vi "IsEmptyNextRecordListCtrl.vi"(11 "testcaseList":refnum<vi>) -> (3 "is empty?":bool)   [LabVIEW 2018, in "Library-Ctrl.lvlib"]
uses:
  Library-Ctrl.lvlib
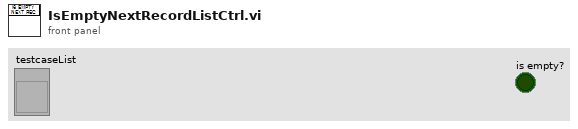
[diagram p1: front panel]
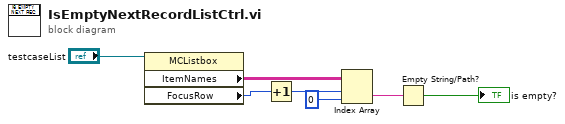
[diagram p0: block diagram]
diagram:
  n1 = property class="MCListbox"(reference="testcaseList") -> ("ItemNames"=w6:string[][], "FocusRow"=w5:i32)  [unwired: 1 in, 2 out]
  n2 = Increment(x=w5) -> (x+1=w4:i32)
  n3 = Index Array(array=w6, index (row)=w4, index (col)=0 ("비활성화된 인덱스 (열)")) -> (element=w2:string)
  n4 = Empty String/Path?(string/path=w2) -> (empty?=→"is empty?":bool)
